vi "Set Template Data.vi"(8 "error in (no error)":errorcluster, 11 "GUI in":refnum<class "GUI.lvclass">) -> (0 "error out":errorcluster, 3 "GUI out":refnum<class "GUI.lvclass">)   [LabVIEW 2020, in "GUI.lvlib" / "GUI.lvclass"]
uses:
  GUI.lvclass
  C:/Program Files/National Instruments/LabVIEW 2020/vi.lib/ActorFramework/Actor/Actor.lvclass
  <vilib>/ActorFramework/Message Enqueuer/Message Enqueuer.lvclass
  <vilib>/ActorFramework/Actor/Actor.lvclass/Actor.ctl
  <vilib>/ActorFramework/Message Enqueuer/Message Enqueuer.lvclass/Message Enqueuer.ctl
  GUI.lvclass/GUI.ctl
  NI Force Task Messages/Update Template Graph Msg/Update Template Graph Msg.lvclass/Update Template Graph Msg.ctl
  <vilib>/ActorFramework/Message Enqueuer/Init from Existing Queue.vi
  <vilib>/ActorFramework/Message Enqueuer/Enqueue.vi
  NI Force Task Messages/Update Template Graph Msg/Update Template Graph Msg.lvclass
  C:/Program Files/National Instruments/LabVIEW 2020/vi.lib/ActorFramework/Message/Message.lvclass
  <vilib>/ActorFramework/Message Priority Queue/Priority Enqueue.vi
  <vilib>/ActorFramework/Actor/Actor.lvclass
panel:
  out "error out 3":errorcluster
  out "Self Enqueuer":refnum<class "Message Enqueuer.lvclass">
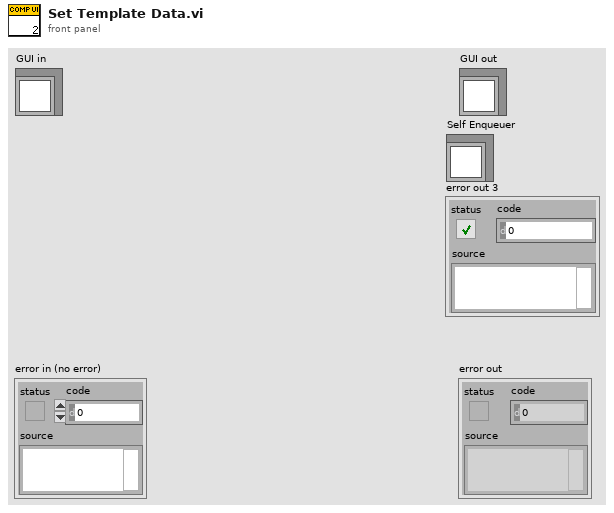
[diagram p1: front panel]
types:
  T1 = typedef "Task info df.ctl" = cluster{"Number of Trials":u8, "Sampling Rate (Hz)":u16, "Trial Duration (s)":u8, "Adjusted MVC (N)":dbl, "R Phase":i32, "L Phase":i32, "L Pattern":u8, "R Pattern":u8, "Time Between Trials (s)":u8, "Lissajous Speed":u16}
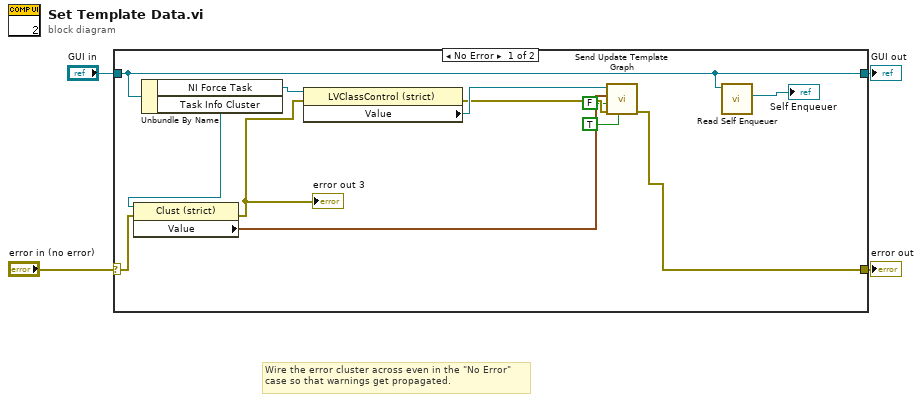
[diagram p0: block diagram]
diagram:
  # "Wire the error cluster across even in the \"No Error\"\ncase so that warnings get propagated."
  n1 = case shown="No Error" "error in (no error)" {
    selector: "error in (no error)" -> [w8 w18]
    tunnel: [w9 w18] -> w3
    tunnel: [w14 w17] -> w1
    tunnel: "GUI in" -> [w14 w17]
    frame No Error {
      n2 = Unbundle By Name(w14) -> ("NI Force Task"=w12:refnum<vi>, "Task Info Cluster"=w15:refnum<vi>)
      n3 = property class="Clust (strict)"(reference=w15, error in=w8) -> (error out=w7:errorcluster, "Value"=w16:T1)  [unwired: 1 out]
      "error out 3" <- w7
      n4 = property class="LVClassControl (strict)"(reference=w12, error in=w7) -> (error out=w10:errorcluster, "Value"=w11:refnum<class "Message Enqueuer.lvclass">)  [unwired: 1 out]
      n5 = call "Send Update Template Graph.vi"("Set Task Info?"=TRUE, "error in (no error)"=w10, "Update Axes Scale"=FALSE, "Task Info In"=w16, "Message Enqueuer in"=w11) -> ("error out"=w9:errorcluster)  [unwired: 5 in, 1 out]
      n6 = call <vilib>:"Read Self Enqueuer.vi"("Actor"=w14) -> ("Self Enqueuer"=→"Self Enqueuer":refnum<class "Message Enqueuer.lvclass">)  [unwired: 10 in]
    }
    frame Error {
    }
  }
  "error out" <- w3
  "GUI out" <- w1
